vi "LVDT Simulation RtDmap.vi"() -> ()   [LabVIEW 8.6]
uses:
  vi.lib/UeiDaq/UeiDaqReadOneScaledScan.vi
  vi.lib/UeiDaq/UeiDaqWriteOneScaledScan.vi
  vi.lib/UeiDaq/UeiDaqCreateLVDTSession.vi
  vi.lib/UeiDaq/UeiDaqCreateSimulatedLVDTSession.vi
  vi.lib/UeiDaq/UeiDaqConfigureTimingForRTDMapIO.vi
panel:
  in  "Excitation frequency":dbl
  in  "Excitation amplitude":dbl
  in  "Sensor Sensitivity":dbl
  in  "Wiring Scheme":enum16{"Four Wires", "Five wires"}(ring)
  in  "Simulated LVDT position":dbl(slide)
  in  "Simulated LVDT Output Resource":string
  out "Measured LVDT position":dbl[][](graph)
  in  "Refresh rate (Hz)":u32
  in  "stop":bool
  in  "LVDT Input Resource":string
  # "LVDT Simulation"
  # "This example takes advantage of the LVDT simulation capability on the AI-254.It Simulates a LVDT out of channel 1 and measures it back on channel 0. You need to connect the folowing pins:\nCh0 S1- <--> Ch1 P1-\nCh0 S1+ <--> Ch1 P1+\nCh0 S2- <--> Ch1 P2-\nCh0 S2+ <--> Ch1 P2+\nCh0 P1- <--> Ch1 S1-\nCh0 P1+ <--> Ch1 S1+\nCh1 S2- <--> Ch1 S2+"
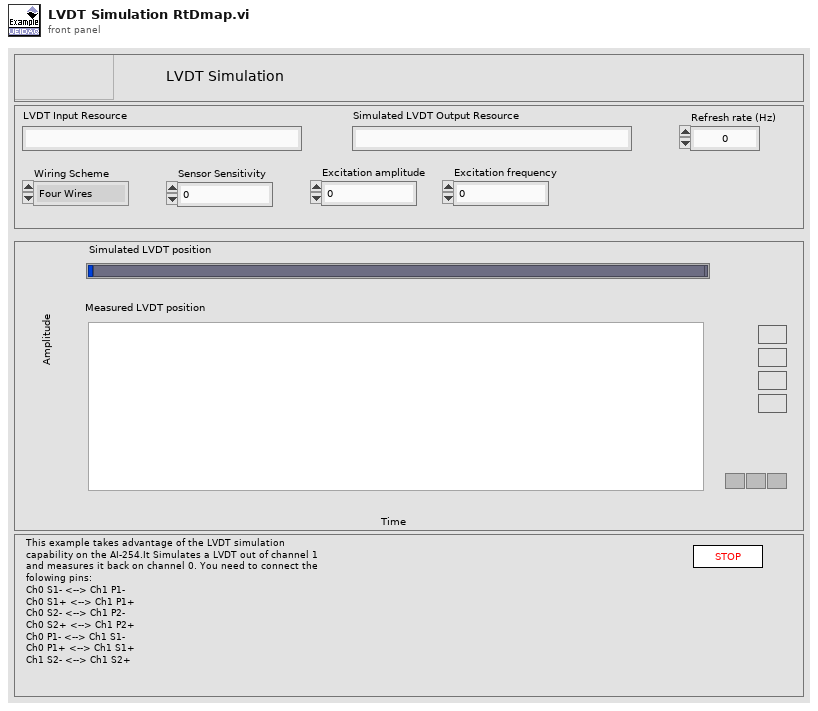
[diagram p1: front panel]
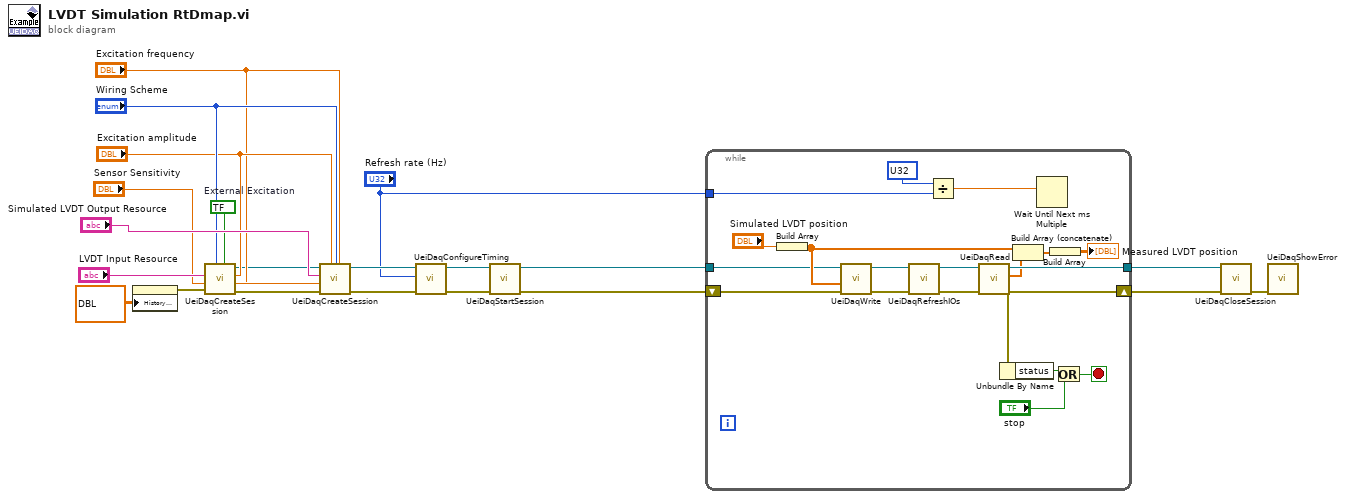
[diagram p0: block diagram]
diagram:
  w12 = bool ?  # External Excitation
  n1 = property on="Measured LVDT position" class="WFChart (strict)"("History Data"=dbl[][] ?) -> (error out=w14:errorcluster)  [unwired: 2 in, 1 out]
  n2 = call-poly "UeiDaqCreateSession.vi"("Excitation frequency"="Excitation frequency", "Excitation voltage"="Excitation amplitude", "External Excitation"=w12, "Wiring Scheme"="Wiring Scheme", "error in (no error)"=w14, "Sensor Sensitivity"="Sensor Sensitivity", "Resource"="LVDT Input Resource") -> ("error out"=w1:errorcluster, "UeiDaq Refnum Out"=w2:refnum<k20>)  [unwired: 3 in]
  n3 = call-poly "UeiDaqCreateSession.vi"("Excitation frequency"="Excitation frequency", "Excitation voltage"="Excitation amplitude", "Wiring Scheme"="Wiring Scheme", "error in (no error)"=w1, "Sensor Sensitivity"="Sensor Sensitivity", "Resource"="Simulated LVDT Output Resource", "UeiDaq Refnum In"=w2) -> ("error out"=w20:errorcluster, "UeiDaq Refnum Out"=w21:refnum<k20>)  [unwired: 3 out]
  n4 = call-poly "UeiDaqConfigureTiming.vi"("error in (no error)"=w20, "Rate"="Refresh rate (Hz)", "UeiDaq Refnum In"=w21) -> ("error out"=w7:errorcluster, "UeiDaq Refnum Out"=w5:refnum<k20>)  [unwired: 7 out]
  n5 = call "UeiDaqStartSession.vi"("error in (no error)"=w7, "UeiDaq Refnum In"=w5) -> ("error out"=w3:errorcluster, "UeiDaq Refnum Out"=w8:refnum<k20>)  [unwired: 8 out]
  n6 = while {
    tunnel: w8 -> [w26]
    tunnel: [w38] -> w17
    shift-right: [w35] -> w6
    shift-left: w3 -> [w27]
    tunnel: "Refresh rate (Hz)" -> [w29]
    stop <- w39 stop-if-true
    n7 = Build Array("Simulated LVDT position") -> (w33:dbl[])
    n8 = call-poly "UeiDaqWrite.vi"("error in (no error)"=w27, "Scaled Data"=w33, "UeiDaq Refnum In"=w26) -> ("error out"=w24:errorcluster, "UeiDaq Refnum Out"=w25:refnum<k20>)  [unwired: 1 in, 6 out]
    n9 = call "UeiDaqRefreshIOs.vi"("error in (no error)"=w24, "UeiDaq Refnum In"=w25) -> ("error out"=w22:errorcluster, "UeiDaq Refnum Out"=w23:refnum<k20>)  [unwired: 8 in]
    n10 = Divide(x=u32 ?, y=w29) -> (x/y=w28:dbl)
    n11 = call-poly "UeiDaqRead.vi"("error in (no error)"=w22, "UeiDaq Refnum In"=w23) -> ("error out"=w35:errorcluster, "Scaled Data"=w36:dbl[], "UeiDaq Refnum Out"=w38:refnum<k20>)  [unwired: 7 out]
    n12 = Unbundle By Name(w35) -> ("status"=w37:bool)
    n13 = Build Array (concatenate)(w33, w36) -> (w32:dbl[])
    n14 = Wait Until Next ms Multiple(millisecond multiple=w28) -> ()  [unwired: 1 out]
    n15 = Build Array(w32) -> (→"Measured LVDT position":dbl[][])
    n16 = Or(x=w37, y="stop") -> (x .or. y?=w39:bool)
  }
  n17 = call "UeiDaqCloseSession.vi"("error in (no error)"=w6, "UeiDaq Refnum In"=w17) -> ("error out"=w16:errorcluster)  [unwired: 1 in, 8 out]
  n18 = call "UeiDaqShowError.vi"("error in (no error)"=w16) -> ()  [unwired: 2 in, 9 out]
